vi "Model Initial Values - Import Inport Channel.vi"(4 "Initial Value":dbl, 6 "Inport Name":string, 7 "Overwrite?":bool, 8 "error in":errorcluster, 9 "Inport Ref":T1 format="%.0x", 10 "Inport References":string, 11 "Section Ref":T1 format="%.0x") -> (0 "error out":errorcluster, 1 "Created New?":bool, 2 "Dependent Nodes":T2 {"Inport Refs" format="%.0x"}, 3 "Section Ref out":T1 format="%.0x")   [LabVIEW 2011, in "Model Initial Values Custom Device.lvlib"]
uses:
  Model Initial Values Custom Device.lvlib
  <vilib>/NI Veristand/Custom Device API/Custom Device Item Ref.ctl
  Model Initial Values - Global.vi
  <vilib>/NI Veristand/Custom Device API/Set Item Property (String Array).vi
  <vilib>/NI Veristand/Custom Device API/Set Item Property (Double Array).vi
  <vilib>/NI Veristand/Custom Device API/Custom Device API.lvlib
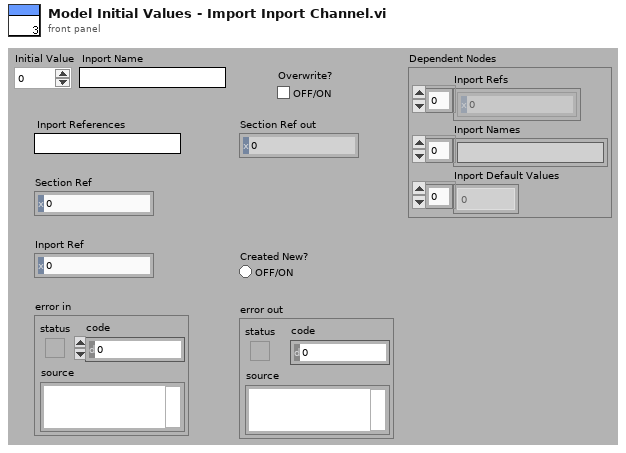
[diagram p1: front panel]
types:
  T1 = typedef "Custom Device API.lvlib/Custom Device Item Ref.ctl" = u64
  T2 = cluster{"Inport Refs":T1[], "Inport Names":string[], "Inport Default Values":dbl[]}
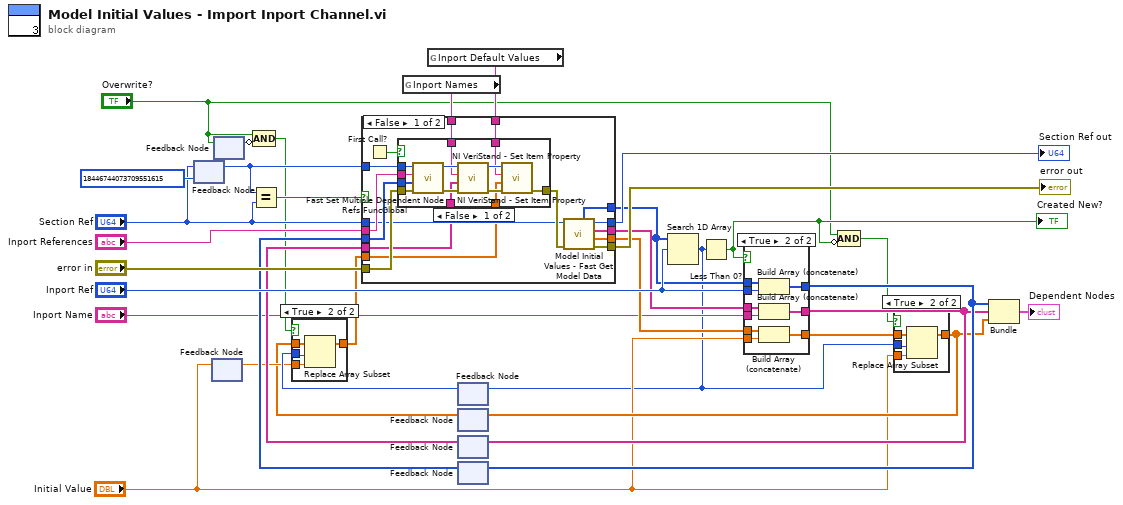
[diagram p0: block diagram]
diagram:
  n1 = feedback-in #1("Section Ref") -> ()
  n2 = feedback #1(T1 18446744073709551615 ("Section Ref")) -> (w23:T1)
  n3 = feedback #2() -> (w6:dbl)  [unwired: 1 in]
  n4 = feedback-in #2("Initial Value") -> ()
  n5 = feedback #3() -> (w10:bool)  [unwired: 1 in]
  n6 = feedback-in #3("Overwrite?") -> ()
  n7 = Equal?(x=w23, y="Section Ref") -> (x = y?=w26:bool)
  n8 = Compound Arithmetic op=AND("Overwrite?", invert w10) -> (w8:bool)
  n9 = global read "Model Initial Values - Global.vi" "Inport Names"() -> (w14:string)
  n10 = global read "Model Initial Values - Global.vi" "Inport Default Values"() -> (w13:string)
  n11 = feedback #4() -> (w7:i32)  [unwired: 1 in]
  n12 = feedback #5() -> (w2:dbl[])  [unwired: 1 in]
  n13 = case shown="True" w8 {
    tunnel: w2 -> [w34 w38]
    tunnel: [w34 w37] -> w1
    tunnel: w6 -> [_ w36]
    tunnel: w7 -> [_ w35]
    frame False {
    }
    frame True {
      n14 = Replace Array Subset(array=w38, new element=w36, index=w35) -> (w37:dbl[])
    }
  }
  n15 = feedback #6() -> (w20:string[])  [unwired: 1 in]
  n16 = feedback #7() -> (w24:T1[])  [unwired: 1 in]
  n17 = case shown="False" w26 {
    tunnel: "Inport References" -> [w53 _]
    tunnel: [w46 w73] -> w32
    tunnel: [w47 w71] -> w25
    tunnel: [w48 w72] -> w31
    tunnel: "error in" -> [w50 w72]
    tunnel: "Section Ref" -> [w45 w73]
    tunnel: w24 -> [w51 w71]
    tunnel: w23 -> [w52 _]
    tunnel: [w44 w70] -> w22
    tunnel: [w43 w69] -> w21
    tunnel: w20 -> [w42 w70]
    tunnel: w1 -> [w41 w69]
    tunnel: w14 -> [w40 _]
    tunnel: w13 -> [w39 _]
    frame False {
      n18 = First Call?() -> (First Call?: T/F=w54:bool)
      n19 = case shown="False" w54 {
        tunnel: w52 -> [w67 _]
        tunnel: w53 -> [w66 _]
        tunnel: w51 -> [w65 _]
        tunnel: w50 -> [w64 w68]
        tunnel: [w59 w68] -> w49
        tunnel: w42 -> [w61 _]
        tunnel: w41 -> [w57 _]
        tunnel: w40 -> [w56 _]
        tunnel: w39 -> [w55 _]
        frame False {
          n20 = call "Fast Set Multiple Dependent Node Refs FuncGlobal.vi"("error in (no error)"=w64, "Dependent Node Refs"=w65, "Base Property Name"=w66, "Item Ref in"=w67) -> ("error out"=w63:errorcluster, "Item Ref out"=w62:T1)  [unwired: 6 in]
          n21 = call-poly <vilib>:"NI VeriStand - Set Item Property.vi"("error in (no error)"=w63, "Value"=w61, "Property Name"=w56, "Item Ref in"=w62) -> ("error out"=w60:errorcluster, "Item Ref out"=w58:T1)  [unwired: 5 in, 1 out]
          n22 = call-poly <vilib>:"NI VeriStand - Set Item Property.vi"("error in (no error)"=w60, "Value"=w57, "Property Name"=w55, "Item Ref in"=w58) -> ("error out"=w59:errorcluster)  [unwired: 5 in, 2 out]
        }
        frame True {
        }
      }
      n23 = call "Model Initial Values - Fast Get Model Data.vi"("error in (no error)"=w49, "Local Model Ref in"=w45) -> ("error out"=w48:errorcluster, "Inport Default Values"=w43:dbl[], "Inport Names"=w44:string[], "Local Model Ref out"=w46:T1, "Inport Refs"=w47:T1[])  [unwired: 4 in, 1 out]
    }
    frame True {
    }
  }
  "Section Ref out" <- w32
  "error out" <- w31
  n24 = Search 1D Array(1D array=w25, element="Inport Ref") -> (index of element=w4:i32)  [unwired: 1 in]
  n25 = feedback-in #4(w4) -> ()
  n26 = Less Than 0?(x=w4) -> (x < 0?=w11:bool)
  "Created New?" <- w11
  n27 = case shown="True" w11 {
    tunnel: [w76 w85] -> w18
    tunnel: w25 -> [w76 w84]
    tunnel: "Inport Ref" -> [_ w83]
    tunnel: w22 -> [w75 w82]
    tunnel: w21 -> [w74 w81]
    tunnel: [w74 w80] -> w3
    tunnel: [w75 w79] -> w17
    tunnel: "Inport Name" -> [_ w78]
    tunnel: "Initial Value" -> [_ w77]
    frame False {
    }
    frame True {
      n28 = Build Array (concatenate)(w84, w83) -> (w85:T1[])
      n29 = Build Array (concatenate)(w82, w78) -> (w79:string[])
      n30 = Build Array (concatenate)(w81, w77) -> (w80:dbl[])
    }
  }
  n31 = feedback-in #6(w17) -> ()
  n32 = feedback-in #7(w18) -> ()
  n33 = Compound Arithmetic op=AND("Overwrite?", invert w11) -> (w12:bool)
  n34 = case shown="True" w12 {
    tunnel: w3 -> [w86 w90]
    tunnel: [w86 w89] -> w15
    tunnel: "Initial Value" -> [_ w88]
    tunnel: w4 -> [_ w87]
    frame False {
    }
    frame True {
      n35 = Replace Array Subset(array=w90, new element=w88, index=w87) -> (w89:dbl[])
    }
  }
  n36 = feedback-in #5(w15) -> ()
  n37 = Bundle("Inport Refs"=w18, "Inport Names"=w17, "Inport Default Values"=w15) -> (→"Dependent Nodes":T2)  [unwired: 1 in]
